vi "JL_APLPath.vi"(8 "Error In":errorcluster, 9 "APL Search String":T1(ring), 11 "Folder Path":path=path "\\\\itnas.appl.ge.com\\technology/Electronics/InProcess/Software/ci_builds/JusticeLeague_Develop") -> (0 "Error Out":errorcluster, 1 "Report text":string, 2 "Found ?":bool, 3 "File Path":path=path "\\\\itnas.appl.ge.com\\technology/Electronics/InProcess/Software/ci_builds/2015_VA_Washer/2015-03-06_03-42-38(Build-1952)/Binaries/2015VAWasher_Param_QA_Cycle_1_62_99_1.apl")   [LabVIEW 2018]
doc: "This VI will search for the most recent version of software apls and return its path. You can search for various firware or xml apls.\n\nIf not found it will return an empty path, as well and boolean and report text."
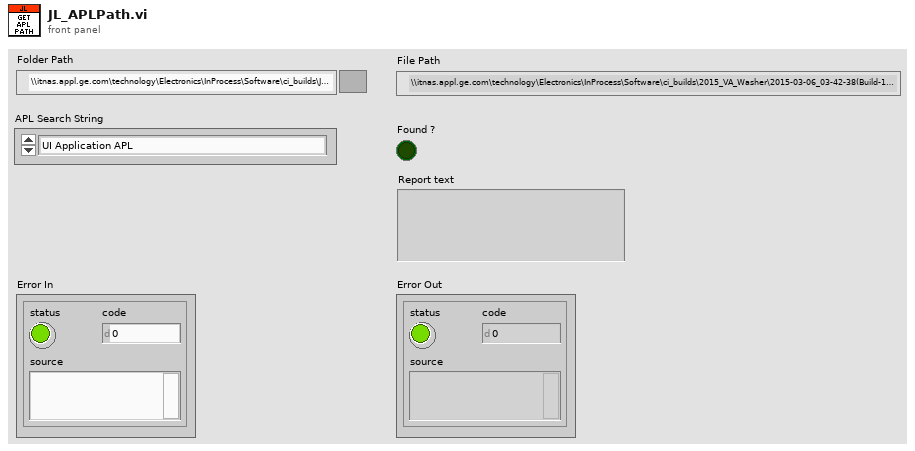
[diagram p1: front panel]
types:
  T1 = enum16{"UI Application APL", "UI Parametric APL", "MC APL", "ERD Definitions XML"}
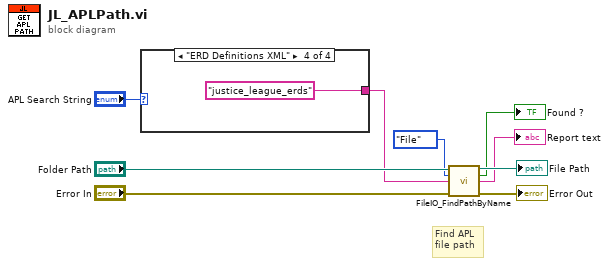
[diagram p0: block diagram]
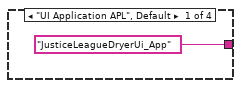
[diagram p2: hidden frame]
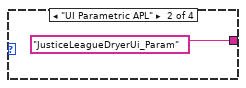
[diagram p3: hidden frame]
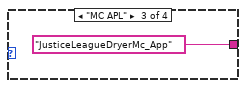
[diagram p4: hidden frame]
diagram:
  # "Find APL\nfile path"
  n1 = case shown="\"ERD Definitions XML\"" "APL Search String" {
    tunnel: ["JusticeLeagueDryerUi_App" "JusticeLeagueDryerUi_Param" "JusticeLeagueDryerMc_App" "justice_league_erds"] -> w5
    frame "UI Application APL", Default {
    }
    frame "UI Parametric APL" {
    }
    frame "MC APL" {
    }
    frame "ERD Definitions XML" {
    }
  }
  n2 = call "FileIO_FindPathByName.vi"("Path In"="Folder Path", "File or Folder ?"=enum16{"Folder", "File"}."File", "File/Folder Search String"=w5, "Error In"="Error In") -> ("Path Out"=→"File Path":path, "Found ?"=→"Found ?":bool, "Report Text"=→"Report text":string, "Error Out"=→"Error Out":errorcluster)  [unwired: 8 in]
